vi "DAQ 1SDI vEPR.vi"() -> ()   [LabVIEW 2013]
uses:
  Strict Type Defs/type_meas_enum.ctl
  <instrlib>/niScope/Controls/niScope vertical coupling.ctl
panel:
  in  "stop":bool
  out "Loop count":i32=4690
  in  "Monitors":enum32{"Monitors On", "Monitors Off"}(tab)
  out "Var(p1+p2)":dbl(graph)=1.0142124161365378
  out "Var(p2+p3)":dbl(graph)=0.6065160666682574
  out "Var(p1+p3)":dbl(graph)=0.5661489724627885
  out "Var(x1-x2)":dbl(graph)=1.0142124161365378
  out "Var(x2-x3)":dbl(graph)=0.6065160666682574
  out "Var(x1-x3)":dbl(graph)=0.5661489724627885
  out "covariance HD 1 & 2":dbl(graph)=0.19831028169384832
  out "Conditional variance HD 1|2":dbl(graph)=1.0142124161365378
  out "Conditional variance HD 1|3":dbl(graph)=0.6065160666682574
  out "Conditional variance HD 2|3":dbl(graph)=0.5661489724627885
  out "covariance HD 1 & 3":dbl(graph)=-0.6559385878875881
  out "covariance HD 2 & 3":dbl(graph)=-0.6106758756892631
  in  "Settings":enum32{"Settings and Record", "Under the hood"}(tab)=enum."Under the hood"
  in  "Delay timing (ms)":u32(knob)=43 scale=0.0..250.0
  in  "Number of monitor samples":i32=10000 format="%.0p"
  in  "File location":path=path "C:/ni-rt/LabVIEW Data/July1/35dB109"
  in  "Type of measurement":T1=enum."electronic"
  in  "File root name":string="Real"
  in  "Number of samples save":i32=2000000 format="%.0p"
  in  "reset sn":bool
  in  "Shot noise start":bool
  in  "Additional text":string="OPA 1 optical power set to 15mV on HD A.\nOPA 2 optical power set to 15mV on HD B.\nLocal oscillator is set to 5V on HD.\nParametric gain set to 15 for OPA 1.\nParametric gain set to 15 for OPA 2.\nVertical range set to 0.5V for both channels.\nSample rate set to 14MS/s.\nMax input freq set to7MHz.\nVisibility between OPA 1 & OPA 2 = 99.6\nVisibility between OPA 1 & L.O.B = 98.9\nVisibility between OPA 1 & L.O. A = 98.9\nBoth squeezers expected to produce -7dB/11dB.\nLoss on EPR B =55.33% (3.5dB) \n"
  in  "Record":bool
  in  "Number of Files":i32=2
  out "File count":i32=1
  in  "Run":string="9"
  in  "hbar":dbl
  out "Cluster":T2={"Actual samples acquired ch 1"=120000, "Actual samples acquired ch 0"=120000, "Actual samples acquired ch 2"=120000}
  in  "Channel Parms":T4={"Input impedance (Ohms)"=2, "Maximum input frequency (Hz)"=7.0, "vertical coupling"=1, "Probe attenuation"=1.0, "Vertical range (V)"=1.0, "Vertical offset"=0.0, "channel enabled"=TRUE} {"Input impedance (Ohms)" items=["1 mega ohm"=0, "50 ohms"=2]; "Maximum input frequency (Hz)" format="%#_6p"; "vertical coupling" items=["AC", "DC", "Ground"]}
  in  "IIR filter specifications":T5={"Topology"=enum."Butterworth", "Type"=enum."Bandpass", "Order"=6, "Lower Fc"=2900000.0, "Upper Fc"=3100000.0, "PB Ripple"=1.0, "SB Attenuation"=60.0} {"PB Ripple" format="%0.2f"; "SB Attenuation" format="%0.2f"; "Lower Fc" format="%0.2p"; "Upper Fc" format="%0.2p"}
  out "error out":errorcluster caption="error out final"
  in  "max time (s)":dbl=10.0 caption="Time to run (s)"
  in  "Reference position":dbl(slide)=50.0 scale=0.0..100.0
  in  "Minimum sample rate (S/s)":dbl=14000000.0 format="%#_6p"
  out "Video bandwidth (Hz)":dbl=7.0
  in  "DAQ Cards":T6={"DAQ Card 1"="Dev2", "DAQ Card 2"="Dev3"}
  # "Variance won't be displayed until shot noise is taken"
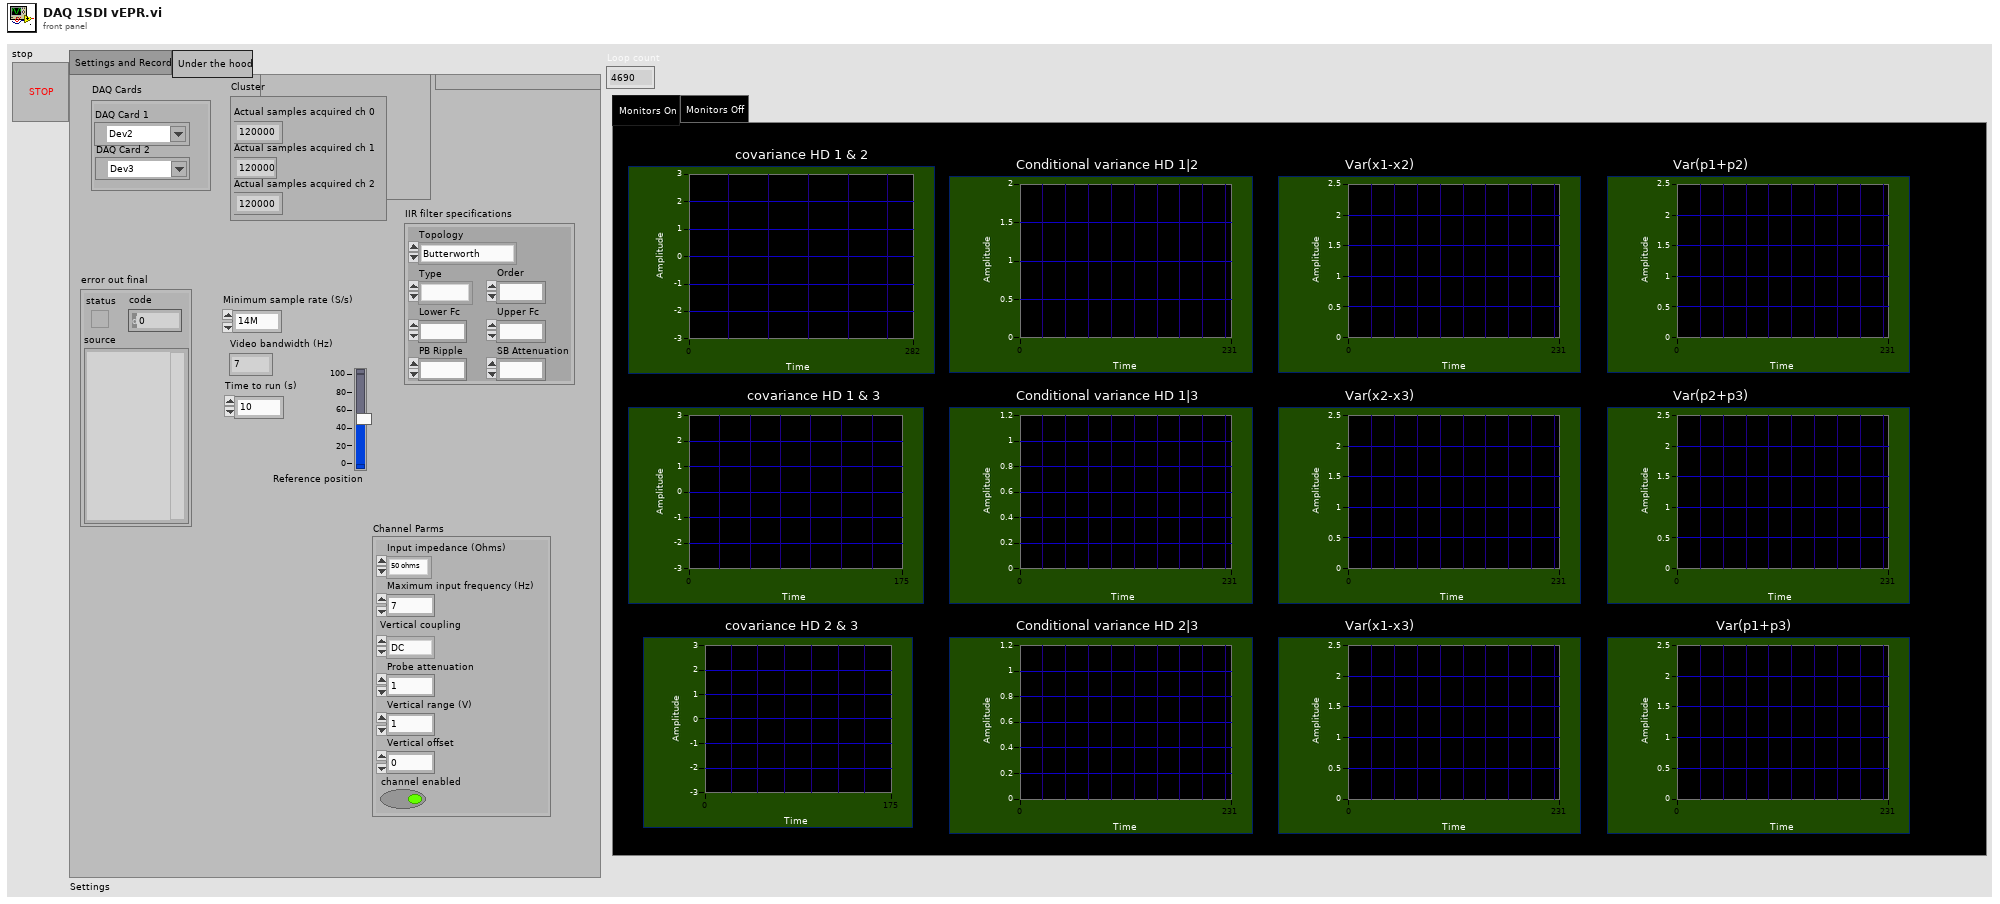
[diagram p1: front panel]
types:
  T1 = typedef "type_meas_enum.ctl" = enum16{"shot", "x", "p", "electronic"}
  T2 = cluster{"Actual samples acquired ch 1":i32, "Actual samples acquired ch 0":i32, "Actual samples acquired ch 2":i32}
  T3 = typedef "niScope vertical coupling.ctl" = i32
  T4 = cluster{"Input impedance (Ohms)":u32, "Maximum input frequency (Hz)":dbl, "vertical coupling":T3, "Probe attenuation":dbl, "Vertical range (V)":dbl, "Vertical offset":dbl, "channel enabled":bool}
  T5 = cluster{"Topology":enum16{"Off", "Butterworth", "Chebyshev", "Inverse Chebyshev", "Elliptic", "Bessel"}, "Type":enum16{"Lowpass", "Highpass", "Bandpass", "Bandstop"}, "Order":i32, "Lower Fc":dbl, "Upper Fc":dbl, "PB Ripple":dbl, "SB Attenuation":dbl}
  T6 = cluster{"DAQ Card 1":refnum<k15>, "DAQ Card 2":refnum<k15>}
  T7 = cluster{"instrument handle":refnum<k15>, "instrument handle":refnum<k15>}
  T8 = cluster{"instrument handle out 0":refnum<k15>, "instrument handle out 1":refnum<k15>}
  T9 = cluster{"actualSamples":i32, "actualSamples":i32, "actualSamples":i32}
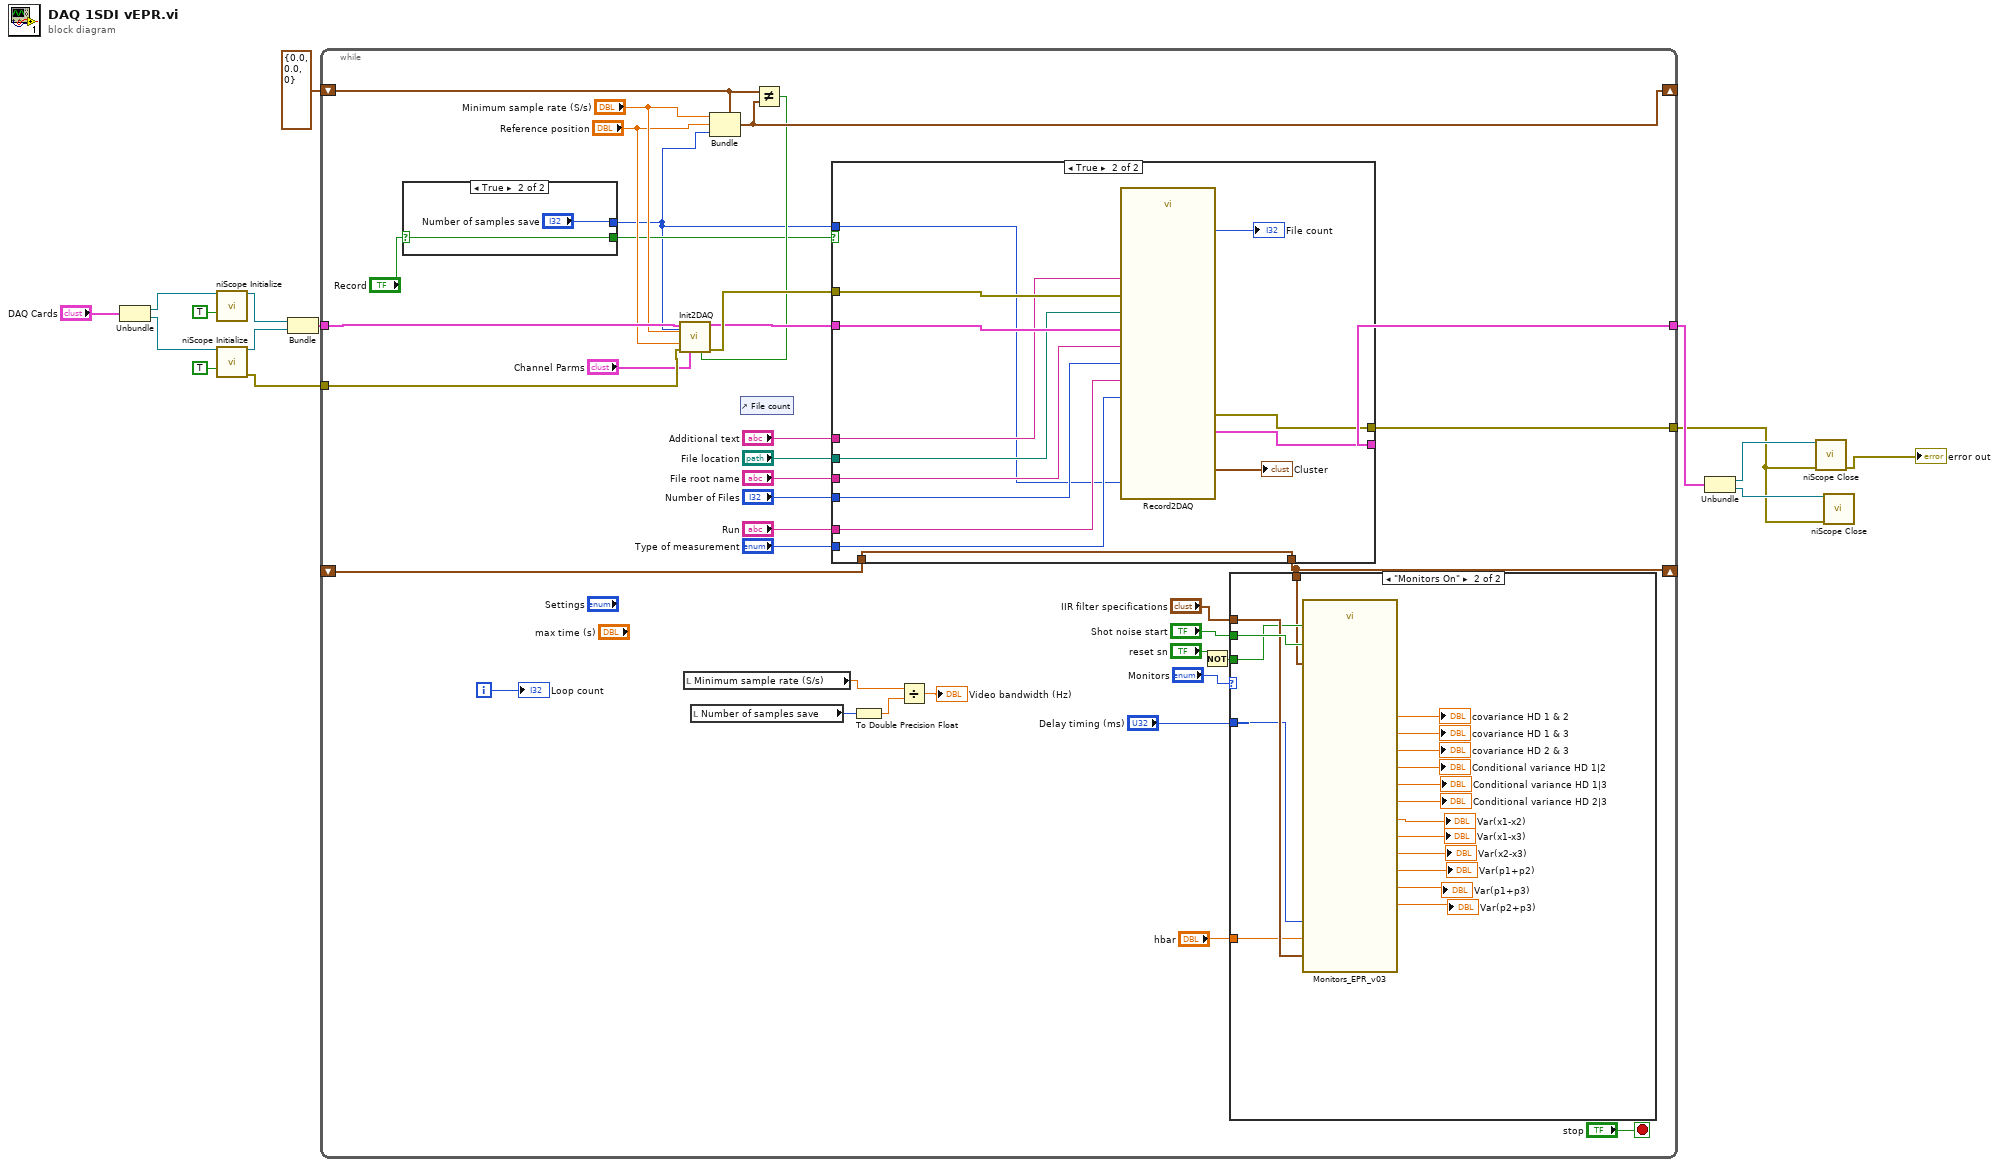
[diagram p0: block diagram]
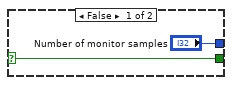
[diagram p2: hidden frame]
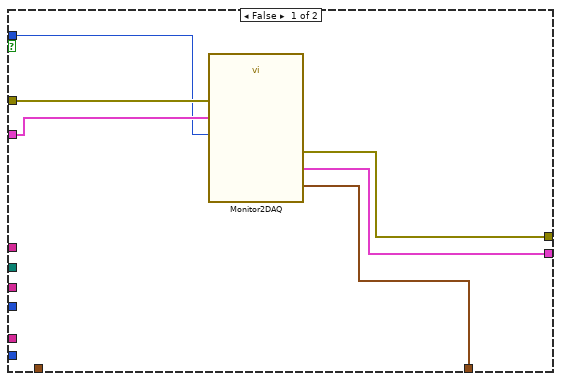
[diagram p4: hidden frame]
diagram:
  n1 = Unbundle("DAQ Cards") -> ("DAQ Card 1"=w7:refnum<k15>, "DAQ Card 2"=w6:refnum<k15>)
  n2 = call <instrlib>:"niScope Initialize.vi"("resource name"=w7, "reset device"=TRUE) -> ("instrument handle"=w4:refnum<k15>)  [unwired: 12 in, 1 out]
  n3 = call <instrlib>:"niScope Initialize.vi"("resource name"=w6, "reset device"=TRUE) -> ("instrument handle"=w3:refnum<k15>, "error out"=w5:errorcluster)  [unwired: 12 in]
  n4 = Bundle("instrument handle"=w4, "instrument handle"=w3) -> (w2:T7)  [unwired: 1 in]
  n5 = while {
    tunnel: [w45] -> w11
    tunnel: w5 -> [w31]
    shift-right: [w26] -> _
    shift-left: cluster{dbl, dbl, i32} {0.0, 0.0, 0} -> [w27]
    shift-right: [w21] -> _
    shift-left: _ -> [w20]
    tunnel: w2 -> [w32]
    tunnel: [w34] -> w15
    i -> [w47]
    stop <- "stop" stop-if-true
    n6 = case shown="True" "Record" {
      selector: "Record" -> [w53 w55]
      tunnel: ["Number of monitor samples" "Number of samples save"] -> w17
      tunnel: [w53 w55] -> w22
      frame False {
      }
      frame True {
      }
    }
    n7 = local read "Minimum sample rate (S/s)"() -> (w35:dbl)
    n8 = local read "Number of samples save"() -> (w37:i32)
    n9 = Bundle(cluster=w27, "Minimum sample rate (S/s)", "Reference position", w17) -> (w26:cluster{dbl, dbl, i32})
    n10 = control-ref of="File count"() -> ()  [unwired: 1 out]
    n11 = Not Equal?(x=w27, y=w26) -> (x != y?=w25:bool)
    n12 = call "Init2DAQ.vi"("resource names"=w32, "min record length"=w17, "min sample rate"="Minimum sample rate (S/s)", "reference position"="Reference position", "error in"=w31, "channel parms"="Channel Parms", "Ch param"=w25) -> ("instrument out"=w33:T8, "error out"=w51:errorcluster)  [unwired: 7 in]
    n13 = case shown="True" w22 {
      tunnel: w33 -> [w78 w93]
      tunnel: w51 -> [w79 w92]
      tunnel: [w77 w91] -> w45
      tunnel: "Additional text" -> [_ w90]
      tunnel: "File location" -> [_ w89]
      tunnel: "File root name" -> [_ w88]
      tunnel: "Number of Files" -> [_ w87]
      tunnel: "Run" -> [_ w86]
      tunnel: "Type of measurement" -> [_ w85]
      tunnel: [w76 w81] -> w21
      tunnel: [w75 w82] -> w34
      tunnel: w20 -> [_ w81]
      tunnel: w17 -> [w74 w80]
      frame False {
        n14 = call "Monitor2DAQ.vi"("instrument in"=w78, "error in"=w79, "numSamples"=w74) -> ("instrument out"=w75:T8, "wfm"=w76:waveform(dbl)[], "error out"=w77:errorcluster)  [unwired: 10 in]
      }
      frame True {
        n15 = call "Record2DAQ.vi"("instrument in"=w93, "Additional text"=w90, "numSamples"=w80, "File location"=w89, "Type of\nmeasurement"=w85, "Name root"=w88, "error in"=w92, "Run"=w86, "number of files"=w87) -> ("output cluster"=→"Cluster":T9, "instrument out"=w82:T8, "File count"=→"File count":i32, "error out"=w91:errorcluster)  [unwired: 2 in, 1 out]
      }
    }
    n16 = To Double Precision Float(number=w37) -> (double precision float=w36:dbl)
    n17 = Divide(x=w35, y=w36) -> (x/y=→"Video bandwidth (Hz)":dbl)
    n18 = Not(x="reset sn") -> (.not. x?=w30:bool)
    n19 = case shown="\"Monitors On\"" "Monitors" {
      tunnel: "Shot noise start" -> [_ w73]
      tunnel: "IIR filter specifications" -> [_ w72]
      tunnel: w30 -> [_ w71]
      tunnel: w21 -> [_ w70]
      tunnel: "Delay timing (ms)" -> [_ w63]
      tunnel: "hbar" -> [_ w59]
      frame "Monitors Off" {
      }
      frame "Monitors On" {
        n20 = call "Monitors_EPR_v03.vi"("IIR filter specifications"=w72, "reset SN"=w71, "Shot noise start"=w73, "wfm"=w70, "hbar"=w59, "Wait(mSec)"=w63) -> ("Var(p1+p3)"=→"Var(p1+p3)":dbl, "Var(p2+p3)"=→"Var(p2+p3)":dbl, "Var(p1+p2)"=→"Var(p1+p2)":dbl, "conditional variance B1|A"=→"Conditional variance HD 2|3":dbl, "covariance B01"=→"covariance HD 1 & 2":dbl, "Var(x1-x2)"=→"Var(x1-x2)":dbl, "covariance B0A"=→"covariance HD 1 & 3":dbl, "covariance B1A"=→"covariance HD 2 & 3":dbl, "Var(x2-x3)"=→"Var(x2-x3)":dbl, "conditional variance B0|1"=→"Conditional variance HD 1|2":dbl, "conditional variance B0|A"=→"Conditional variance HD 1|3":dbl, "Var(x1-x3)"=→"Var(x1-x3)":dbl)  [unwired: 10 in]
      }
    }
    "Loop count" <- w47
  }
  n21 = Unbundle(w15) -> ("instrument handle out 0"=w14:refnum<k15>, "instrument handle out 1"=w13:refnum<k15>)
  n22 = call <instrlib>:"niScope Close.vi"("instrument handle"=w14, "error in"=w11) -> ("error out"=→"error out":errorcluster)  [unwired: 13 in]
  n23 = call <instrlib>:"niScope Close.vi"("instrument handle"=w13, "error in"=w11) -> ()  [unwired: 13 in, 1 out]
